vi "Normalize Coordinates2.vi"(9 "Camera Type":T1, 10 "Targets":T4(array[cluster]), 11 "Image in":T5) -> (2 "Found Totes":T2(array[cluster]) {"Normalized Rect"."Numeric 5" format="%#_2g"; "Normalized Rect"."Numeric 3" format="%#_2g"; "Normalized Rect"."Numeric 2" format="%#_2g"; "Normalized Rect"."Numeric" format="%#_2g"}, 3 "Sorted Scores":T3(array[cluster]) {"Correlation" format="%#_3g"; "Scale" format="%#_3g"; "Score" format="%#_3g"})   [LabVIEW 2014]
doc: "Normalize the rectangle and center so that they range from -1 to 1, left to right and bottom to top. This helps with producing joystick coordinates for driving the robot."
uses:
  <vilib>/vision/Image Controls.llb/IMAQ Image.ctl
  Camera Types.ctl
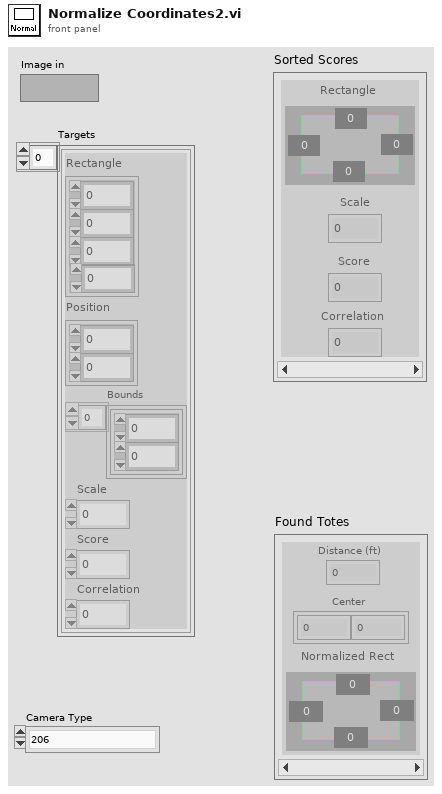
[diagram p1: front panel]
types:
  T1 = typedef "Camera Types.ctl" = enum16{"206", "1011", "1013", "MS HD3000 square", "MS HD3000 640x480"}
  T2 = cluster{"Distance (ft)":dbl, "Center":cluster{dbl, dbl}, "Normalized Rect":cluster{"Numeric":dbl, "Numeric 2":dbl, "Numeric 3":dbl, "Numeric 5":dbl}}[]
  T3 = cluster{"Rectangle":cluster{"Numeric":dbl, "Numeric 2":dbl, "Numeric 3":dbl, "Numeric 5":dbl}, "Scale":dbl, "Score":dbl, "Correlation":dbl}[]
  T4 = cluster{"Rectangle":cluster{"Numeric":dbl, "Numeric 2":dbl, "Numeric 3":dbl, "Numeric 5":dbl}, "Position":cluster{"Numeric":dbl, "Numeric 2":dbl}, "Bounds":cluster{"Numeric":dbl, "Numeric 2":dbl}[], "Scale":dbl, "Score":dbl, "Correlation":dbl}[]
  T5 = typedef "IMAQ Image.ctl" = refnum<image>
  T6 = cluster{"X Resolution":i32, i32, "X Resolution":i32, i32}
  T7 = cluster{"[0]":dbl, "[1]":dbl, "[2]":dbl, "[3]":dbl}
  T8 = cluster{"Numeric":dbl, "Numeric 2":dbl, "Numeric 3":dbl, "Numeric 5":dbl}
  T9 = cluster{"Rectangle":cluster{"Numeric":dbl, "Numeric 2":dbl, "Numeric 3":dbl, "Numeric 5":dbl}, "Scale":dbl, dbl, dbl}
  T10 = cluster{"Distance (ft)":dbl, cluster{dbl, dbl}, cluster{dbl, dbl, dbl, dbl}}
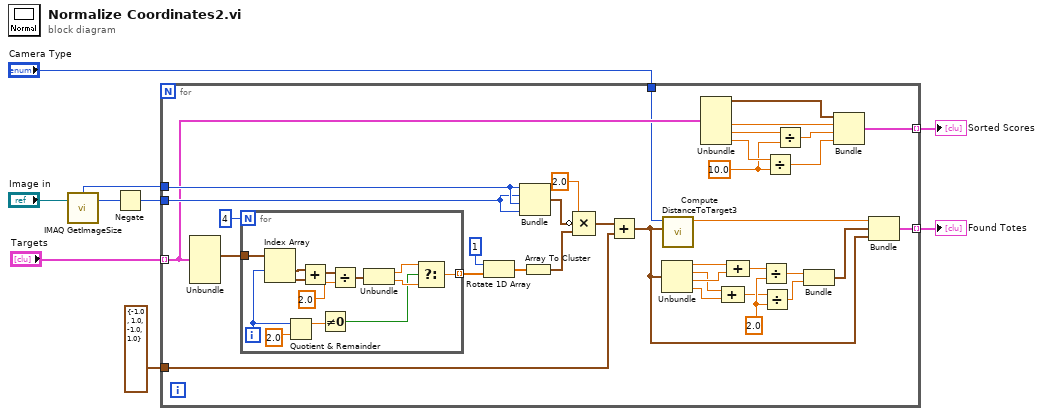
[diagram p0: block diagram]
diagram:
  n1 = call "IMAQ GetImageSize"("Image"="Image in") -> ("Y Resolution"=w7:i32, "X Resolution"=w8:i32)  [unwired: 3 in, 1 out]
  n2 = Negate(x=w7) -> (-x=w9:i32)
  n3 = for {
    tunnel: "Targets" -> [w27] mode=indexing
    tunnel: w9 -> [w43]
    tunnel: w8 -> [w44]
    tunnel: [w30] -> w4 mode=indexing
    tunnel: [w24] -> w1 mode=indexing
    tunnel: cluster{dbl, dbl, dbl, dbl} {-1.0, 1.0, -1.0, 1.0} ("y") -> [w28]
    tunnel: "Camera Type" -> [w18]
    w19 = 10.0
    w35 = 2.0
    n4 = Unbundle(w27) -> ("Bounds"=w15:cluster{"Numeric":dbl, "Numeric 2":dbl}[])  [unwired: 5 out]
    n5 = for {
      N: 4 -> [_]
      tunnel: w15 -> [w57]
      tunnel: [w45] -> w11 mode=indexing
      i -> [w49]
      n6 = Index Array(array=w57, index #1=w49) -> (element #1=w56:cluster{"Numeric":dbl, "Numeric 2":dbl}, element #2=w55:cluster{"Numeric":dbl, "Numeric 2":dbl})  [unwired: 1 in]
      n7 = Quotient & Remainder(x=w49, y=2.0) -> (x-y*floor(x/y)=w47:dbl)  [unwired: 1 out]
      n8 = Add(x=w56, y=w55) -> (x+y=w54:cluster{"Numeric":dbl, "Numeric 2":dbl})
      n9 = Not Equal To 0?(x=w47) -> (x != 0?=w46:bool)
      n10 = Divide(x=w54, y=2.0) -> (x/y=w52:cluster{"Numeric":dbl, "Numeric 2":dbl})
      n11 = Unbundle(w52) -> ("Numeric"=w51:dbl, "Numeric 2"=w50:dbl)
      n12 = Select(t=w51, s=w46, f=w50) -> (s? t:f=w45:dbl)
    }
    n13 = Rotate 1D Array(1:w11, 2:1) -> (0:w12:dbl[])
    n14 = Bundle("X Resolution"=w44, w43, "X Resolution"=w44, w43) -> (w42:T6)  [unwired: 1 in]
    n15 = Array To Cluster(array=w12) -> (cluster=w13:T7)
    n16 = Compound Arithmetic op=MULTIPLY(2.0, invert w42, w13) -> (w41:cluster{dbl, dbl, dbl, dbl})
    n17 = Add(x=w41, y=w28) -> (x+y=w17:cluster{dbl, dbl, dbl, dbl})
    n18 = Unbundle(w17) -> (w39:dbl, w36:dbl, w38:dbl, w37:dbl)
    n19 = call "Compute DistanceToTarget3.vi"("Norm Rect"=w17, "Camera Type"=w18) -> ("Distance (ft)"=w16:dbl)  [unwired: 9 in]
    n20 = Unbundle(w27) -> ("Rectangle"=w25:T8, "Scale"=w26:dbl, "Score"=w20:dbl, "Correlation"=w23:dbl)  [unwired: 2 out]
    n21 = Compound Arithmetic op=ADD(w36, w37) -> (w33:dbl)
    n22 = Compound Arithmetic op=ADD(w39, w38) -> (w34:dbl)
    n23 = Divide(x=w34, y=w35) -> (x/y=w32:dbl)
    n24 = Divide(x=w33, y=w35) -> (x/y=w31:dbl)
    n25 = Divide(x=w23, y=w19) -> (x/y=w22:dbl)
    n26 = Divide(x=w20, y=w19) -> (x/y=w21:dbl)
    n27 = Bundle(w32, w31) -> (w29:cluster{dbl, dbl})  [unwired: 1 in]
    n28 = Bundle("Rectangle"=w25, "Scale"=w26, w21, w22) -> (w24:T9)  [unwired: 1 in]
    n29 = Bundle("Distance (ft)"=w16, w29, w17) -> (w30:T10)  [unwired: 1 in]
  }
  "Sorted Scores" <- w1
  "Found Totes" <- w4
